vi "ArdnoFlush.vi"(7 "Open?":bool, 8 "error in (no error)":errorcluster, 9 "Single / Multivalve?":bool, 10 "Channel":u32, 11 "LINX Resource":T1={"IO"=enum."Remote", "Interface"=enum."Serial", "LINX Device Config"={"Interface"=enum."Serial", "COM Port"="COM13", "TCP Configuration"={"IP Address"="", "Port"=0}, "Device Family"=1, "Device ID"=1, "Device Name"="myRIO-1900", "TCP Ref"=refnum, "Channels"={"DI"=[0, 1, 2, 3, 4, 5, 6, 7, 8, 9, 10, 11, 12, 13, 14, 15, 16, 17, 18, 19, 20, 21, 22, 23, 24, 25, 26, 27, 28, 29, 30, 31, 32, 33, 34, 35, 36, 37, 38, 39, 40, 41, 42, 43, 44, 45, 46], "DO"=[0, 1, 2, 3, 4, 5, 6, 7, 8, 9, 10, 11, 12, 13, 14, 15, 16, 17, 18, 19, 20, 21, 22, 23, 24, 25, 26, 27, 28, 29, 30, 31, 32, 33, 34, 35, 36, 37, 38, 39, 40, 41, 42, 43, 44, 45, 46], "AI"=[0, 1, 2, 3, 4, 5, 6, 7, 8, 9, 10, 11], "AO"=[], "PWM"=[3, 5, 6, 9, 10], "QE"=[], "UART"=[0, 1], "I2C 2"=[0], "SPI"=[0], "CAN"=[], "Servo"=[], "AI Ref (V)"=0.0, "AI Resolution (Bits)"=0, "AO Ref (V)"=0.0, "AO Resolution (Bits)"=0}}}) -> (0 "error out":errorcluster, 3 "LINX Resource out":T1)   [LabVIEW 2018]
uses:
  <vilib>/MakerHub/LINX/Private/Type Defs/LINX Ref.ctl
  <vilib>/MakerHub/LINX/Private/Type Defs/Platform.ctl
  <vilib>/MakerHub/LINX/Private/Type Defs/Interface.ctl
  <vilib>/MakerHub/LINX/Private/Device/Type Defs/LINX Device Config.ctl
  <vilib>/MakerHub/LINX/Private/Device/Type Defs/TCP Config.ctl
  <vilib>/MakerHub/LINX/Private/Device/Type Defs/Channels.ctl
  <vilib>/MakerHub/LINX/Public/Peripherals/Digital/Digital Write N Chans.vi
  <vilib>/MakerHub/LINX/Private/Local IO/LinxDigitalWrite.vi
  <vilib>/MakerHub/LINX/Public/Utilities/Check Channel.vi
  <vilib>/MakerHub/LINX/Private/Utilties/Generate Error.vi
  <vilib>/MakerHub/LINX/LMH-LINX.lvlib
  <vilib>/MakerHub/LINX/Private/Device/Device.lvlib
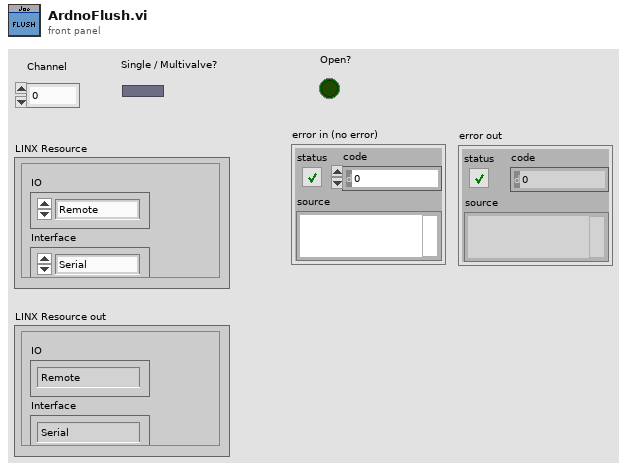
[diagram p1: front panel]
types:
  T1 = typedef "LMH-LINX.lvlib/LINX Ref.ctl" = cluster{"IO":T2, "Interface":T3, "LINX Device Config":T4}
  T2 = typedef "LMH-LINX.lvlib/Platform.ctl" = enum16{"Remote", "Local"}
  T3 = typedef "LMH-LINX.lvlib/Interface.ctl" = enum16{"Serial", "TCP"}
  T4 = typedef "LMH-LINX.lvlib/Device.lvlib/LINX Device Config.ctl" = cluster{"Interface":T3, "COM Port":refnum<visa-resource-name>, "TCP Configuration":T5, "Device Family":u8, "Device ID":u8, "Device Name":string, "TCP Ref":refnum<k5>, "Channels":T6}
  T5 = typedef "LMH-LINX.lvlib/Device.lvlib/TCP Config.ctl" = cluster{"IP Address":string, "Port":u16}
  T6 = typedef "LMH-LINX.lvlib/Channels.ctl" = cluster{"DI":u8[], "DO":u8[], "AI":u8[], "AO":u8[], "PWM":u8[], "QE":u8[], "UART":u8[], "I2C 2":u8[], "SPI":u8[], "CAN":u8[], "Servo":u8[], "AI Ref (V)":dbl, "AI Resolution (Bits)":u8, "AO Ref (V)":dbl, "AO Resolution (Bits)":u8}
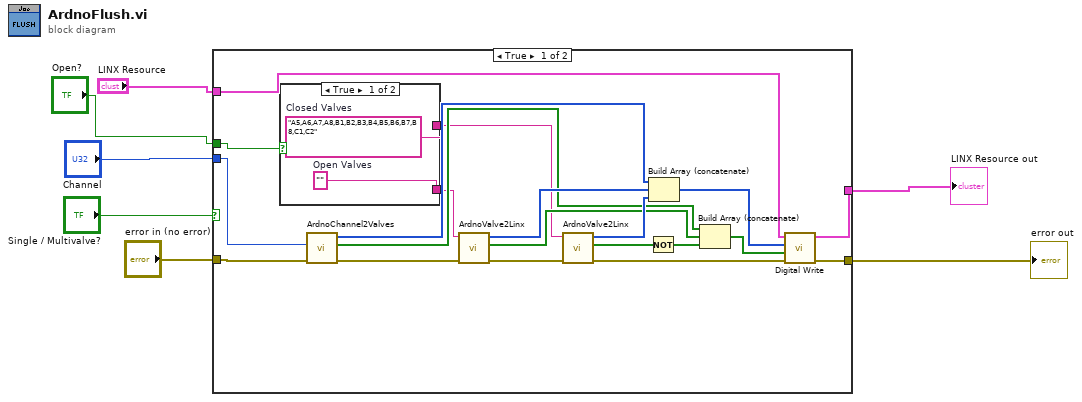
[diagram p0: block diagram]
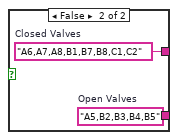
[diagram p2: hidden frame]
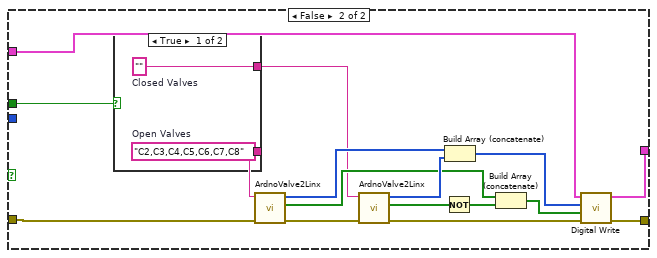
[diagram p3: hidden frame]
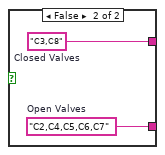
[diagram p4: hidden frame]
diagram:
  n1 = case shown="True" "Single / Multivalve?" {
    tunnel: "error in (no error)" -> [w27 w33]
    tunnel: [w26 w47] -> w6
    tunnel: [w25 w46] -> w5
    tunnel: "Channel" -> [w10 _]
    tunnel: "LINX Resource" -> [w9 w34]
    tunnel: "Open?" -> [w8 w32]
    frame True {
      n2 = case shown="True" w8 {
        tunnel: [w29 w31] -> w12
        tunnel: [w28 w30] -> w11
        frame True {
          w28 = "A5,A6,A7,A8,B1,B2,B3,B4,B5,B6,B7,B8,C1,C2"  # Closed Valves
          w29 = ""  # Open Valves
        }
        frame False {
          w30 = "A6,A7,A8,B1,B7,B8,C1,C2"  # Closed Valves
          w31 = "A5,B2,B3,B4,B5"  # Open Valves
        }
      }
      n3 = call "ArdnoChannel2Valves.vi"("Channel"=w10, "error in (no error)"=w27) -> ("Valve Nums"=w17:i32[], "Valve State"=w16:bool[], "error out"=w15:errorcluster)  [unwired: 6 in]
      n4 = call "ArdnoValve2Linx.vi"("error in (no error)"=w15, "Valve (A1-C8),\n comma separated"=w12) -> ("error out"=w19:errorcluster, "Array"=w21:bool[], "Array 2"=w22:i32[])  [unwired: 7 in]
      n5 = call "ArdnoValve2Linx.vi"("error in (no error)"=w19, "Valve (A1-C8),\n comma separated"=w11) -> ("error out"=w14:errorcluster, "Array"=w24:bool[], "Array 2"=w23:i32[])  [unwired: 7 in]
      n6 = Not(x=w24) -> (.not. x?=w20:bool[])
      n7 = Build Array (concatenate)(w17, w22, w23) -> (w18:i32[])
      n8 = Build Array (concatenate)(w16, w21, w20) -> (w13:bool[])
      n9 = call-poly <vilib>:"Digital Write.vi"("Error In"=w14, "Values"=w13, "DO Channels"=w18, "LINX Resource"=w9) -> ("Error Out"=w26:errorcluster, "LINX Resource"=w25:T1)  [unwired: 6 in]
    }
    frame False {
      n10 = case shown="True" w32 {
        tunnel: [w49 w51] -> w36
        tunnel: [w48 w50] -> w35
        frame True {
          w48 = ""  # Closed Valves
          w49 = "C2,C3,C4,C5,C6,C7,C8"  # Open Valves
        }
        frame False {
          w50 = "C3,C8"  # Closed Valves
          w51 = "C2,C4,C5,C6,C7"  # Open Valves
        }
      }
      n11 = call "ArdnoValve2Linx.vi"("error in (no error)"=w33, "Valve (A1-C8),\n comma separated"=w36) -> ("error out"=w40:errorcluster, "Array"=w42:bool[], "Array 2"=w43:i32[])  [unwired: 7 in]
      n12 = call "ArdnoValve2Linx.vi"("error in (no error)"=w40, "Valve (A1-C8),\n comma separated"=w35) -> ("error out"=w38:errorcluster, "Array"=w45:bool[], "Array 2"=w44:i32[])  [unwired: 7 in]
      n13 = Not(x=w45) -> (.not. x?=w41:bool[])
      n14 = Build Array (concatenate)(w43, w44) -> (w39:i32[])
      n15 = Build Array (concatenate)(w42, w41) -> (w37:bool[])
      n16 = call-poly <vilib>:"Digital Write.vi"("Error In"=w38, "Values"=w37, "DO Channels"=w39, "LINX Resource"=w34) -> ("Error Out"=w47:errorcluster, "LINX Resource"=w46:T1)  [unwired: 6 in]
    }
  }
  "error out" <- w6
  "LINX Resource out" <- w5
